vi "Calculator_multiply-harness.vi"(11 "test case ID":string) -> (3 "result":bool)   [LabVIEW 2018]
doc: "The harness VI is executed for every test case. InstaCoverage passes the test case ID before the execution of the test case in the <b>test case ID</b> input and reads the <b>result</b> output after the execution. If the result is TRUE and no error happens during the execution, then the test case is evaluated as PASSED. If the result is false and no error happens during the execution, then the test case is evaluated as FAILED. Otherwise the test case is evaluated as ERROR.\n\nThe result of the test suite will be PASSED (FAILED) if all (at least one) test cases are PASSED (FAILED). If at least one test case in the test suite has the ERROR result, then the test suite will have ERROR result.\n\n<b>Note: </b>Don't change the connector pane of this VI.\n\nSee the Help Document for more information. (<b>Help</b> > <b>InstaCoverage Help...</b>)"
uses:
  Calculator.lvclass
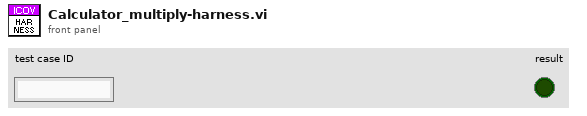
[diagram p1: front panel]
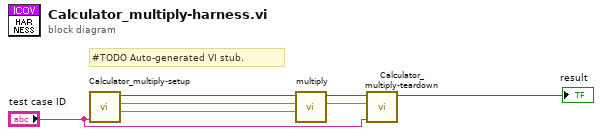
[diagram p0: block diagram]
diagram:
  # "#TODO Auto-generated VI stub."
  n1 = call "Calculator_multiply-setup.vi"("test case ID"="test case ID") -> ("b"=w1:dbl, "a"=w2:dbl, "Calculator in"=w7:refnum<class "Calculator.lvclass">)  [unwired: 8 in]
  n2 = call-dynamic "multiply.vi"("y"=w1, "x"=w2, "Calculator in"=w7) -> ("x*y"=w6:dbl, "Calculator out"=w5:refnum<class "Calculator.lvclass">)  [unwired: 7 in]
  n3 = call "Calculator_multiply-teardown.vi"("test case ID"="test case ID", "x*y"=w6, "Calculator out"=w5) -> ("result"=→"result":bool)  [unwired: 8 in]
